vi "Created.vi"(8 "Alias":string, 9 "Is Priority":bool, 10 "Msg":refnum<class "Msg.lvclass">, 11 "Base Actor in":refnum<class "Base Actor.lvclass">) -> (3 "Base Actor out":refnum<class "Base Actor.lvclass">)   [LabVIEW 2020, in "jettl.lvlib" / "Actor.lvlib" / "Base Actor.lvclass"]
uses:
  Base Actor.lvclass
  Msg/Msg.lvclass
  Relation.ctl
  Attributes/Attributes/Attributes.lvclass
  Error/Error.lvlib
  Actor.lvlib
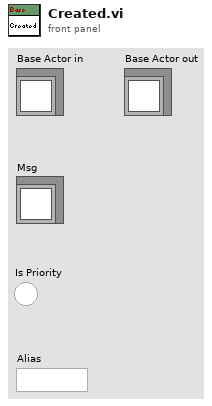
[diagram p1: front panel]
types:
  T1 = typedef "jettl.lvlib/Actor.lvlib/Relation.ctl" = enum16{"Self", "Creator", "Created"}
  T2 = typedef "jettl.lvlib/Actor.lvlib/Msgs.ctl" = set{refnum<class "Msg.lvclass">}
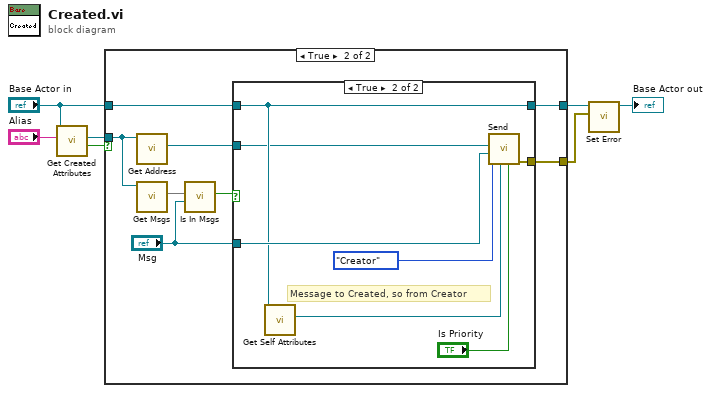
[diagram p0: block diagram]
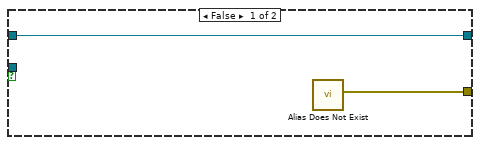
[diagram p2: hidden frame]
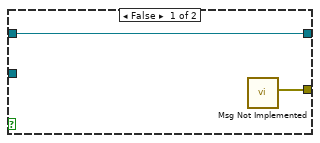
[diagram p3: hidden frame]
diagram:
  n1 = call-dynamic "Get Created Attributes.vi"("Alias"="Alias", "Base Actor in"="Base Actor in") -> ("Is Found"=w2:bool, "Created Attributes"=w1:refnum<class "Attributes.lvclass">)  [unwired: 8 in]
  n2 = case shown="True" w2 {
    tunnel: [w9 w17] -> w5
    tunnel: "Base Actor in" -> [w9 w16]
    tunnel: [w8 w15] -> w3
    tunnel: w1 -> [_ w11]
    frame False {
      n3 = call "Alias Does Not Exist.vi"() -> ("Error"=w8:errorcluster)  [unwired: 11 in]
    }
    frame True {
      n4 = call-dynamic "Get Address.vi"("Attributes in"=w11) -> ("Address"=w12:refnum<user-event>)  [unwired: 10 in]
      n5 = call-dynamic "Get Msgs.vi"("Attributes in"=w11) -> ("Msgs"=w14:T2)  [unwired: 10 in]
      n6 = call "Is In Msgs.vi"("Msg"="Msg", "Msgs"=w14) -> ("Is In Msgs"=w13:bool)  [unwired: 9 in]
      n7 = case shown="True" w13 {
        tunnel: w16 -> [w19 w22]
        tunnel: [w19 w22] -> w17
        tunnel: "Msg" -> [_ w26]
        tunnel: [w18 w21] -> w15
        tunnel: w12 -> [_ w20]
        frame False {
          n8 = call "Msg Not Implemented.vi"() -> ("Error"=w18:errorcluster)  [unwired: 11 in]
        }
        frame True {
          # "Message to Created, so from Creator"
          n9 = call-dynamic "Get Self Attributes.vi"("Base Actor in"=w22) -> ("Self Attributes"=w24:refnum<class "Attributes.lvclass">)  [unwired: 10 in]
          n10 = call "Send.vi"("Is Priority"="Is Priority", "Self Attributes"=w24, "Relation"=Relation."Creator", "Msg"=w26, "Address"=w20) -> ("Error"=w21:errorcluster)  [unwired: 6 in]
        }
      }
    }
  }
  n11 = call-dynamic "Set Error.vi"("Error"=w3, "Base Actor in"=w5) -> ("Base Actor out"=→"Base Actor out":refnum<class "Base Actor.lvclass">)  [unwired: 9 in]
